vi "系统模拟量量化数据解析.vi"(11 "输入字符串":string) -> (3 "系统模拟量量化数据":T1)   [LabVIEW 2016, in "环境动力监测库.lvlib" / "空调库.lvlib"]
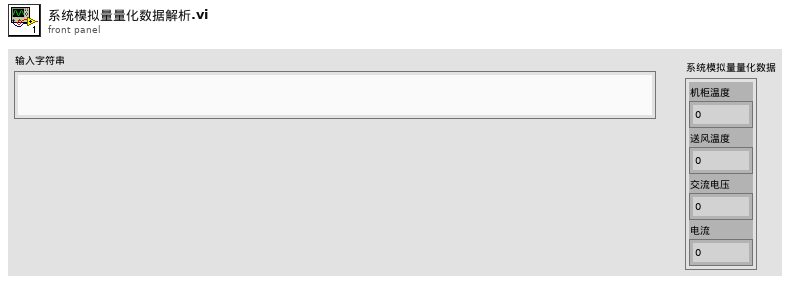
[diagram p1: front panel]
types:
  T1 = cluster{"机柜温度":sgl, "送风温度":sgl, "交流电压":sgl, "电流":sgl}
  T2 = cluster{"机柜温度":u16, "送风温度":u16, "交流电压":u16, "电流":sgl}
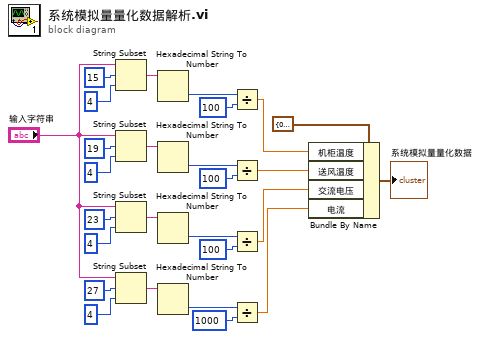
[diagram p0: block diagram]
diagram:
  n1 = String Subset(string="输入字符串", offset (0)=15 ("偏移量(0)"), length (rest)=4 ("长度（剩余）")) -> (substring=w25:string)
  n2 = String Subset(string="输入字符串", offset (0)=19 ("偏移量(0)"), length (rest)=4 ("长度（剩余）")) -> (substring=w22:string)
  n3 = String Subset(string="输入字符串", offset (0)=23 ("偏移量(0)"), length (rest)=4 ("长度（剩余）")) -> (substring=w21:string)
  n4 = String Subset(string="输入字符串", offset (0)=27 ("偏移量(0)"), length (rest)=4 ("长度（剩余）")) -> (substring=w16:string)
  n5 = Hexadecimal String To Number(string=w25) -> (number=w8:u32)  [unwired: 2 in, 1 out]
  n6 = Hexadecimal String To Number(string=w22) -> (number=w7:u32)  [unwired: 2 in, 1 out]
  n7 = Hexadecimal String To Number(string=w21) -> (number=w6:u32)  [unwired: 2 in, 1 out]
  n8 = Hexadecimal String To Number(string=w16) -> (number=w5:u32)  [unwired: 2 in, 1 out]
  n9 = Divide(x=w8, y=u32 100) -> (x/y=w4:dbl)
  n10 = Divide(x=w7, y=u32 100) -> (x/y=w3:dbl)
  n11 = Divide(x=w6, y=u32 100) -> (x/y=w2:dbl)
  n12 = Divide(x=w5, y=u32 1000) -> (x/y=w1:dbl)
  n13 = Bundle By Name(cluster=T2 {"机柜温度"=0, "送风温度"=0, "交流电压"=0, "电流"=0.0} ("系统模拟量量化数据"), "机柜温度"=w4, "送风温度"=w3, "交流电压"=w2, "电流"=w1) -> (→"系统模拟量量化数据":T2)
